vi "decimate cond.vi"(7 "Offset":i32, 8 "error in":errorcluster, 9 "B field array":dbl[](array[numeric]), 10 "Conductance":T1(graph), 11 "Decimation":i32) -> (0 "error out":errorcluster, 2 "decimated B field array":dbl[](array[numeric]), 3 "Decimated conductance":T1(graph))   [LabVIEW 2016, in "Tranconductance SM.lvclass"]
uses:
  Tranconductance SM.lvclass
  <userlib>/_MGI/1D Array/MGI Decimate Array with Offset/MGI Decimate Array with Offset (DBL[]).vi
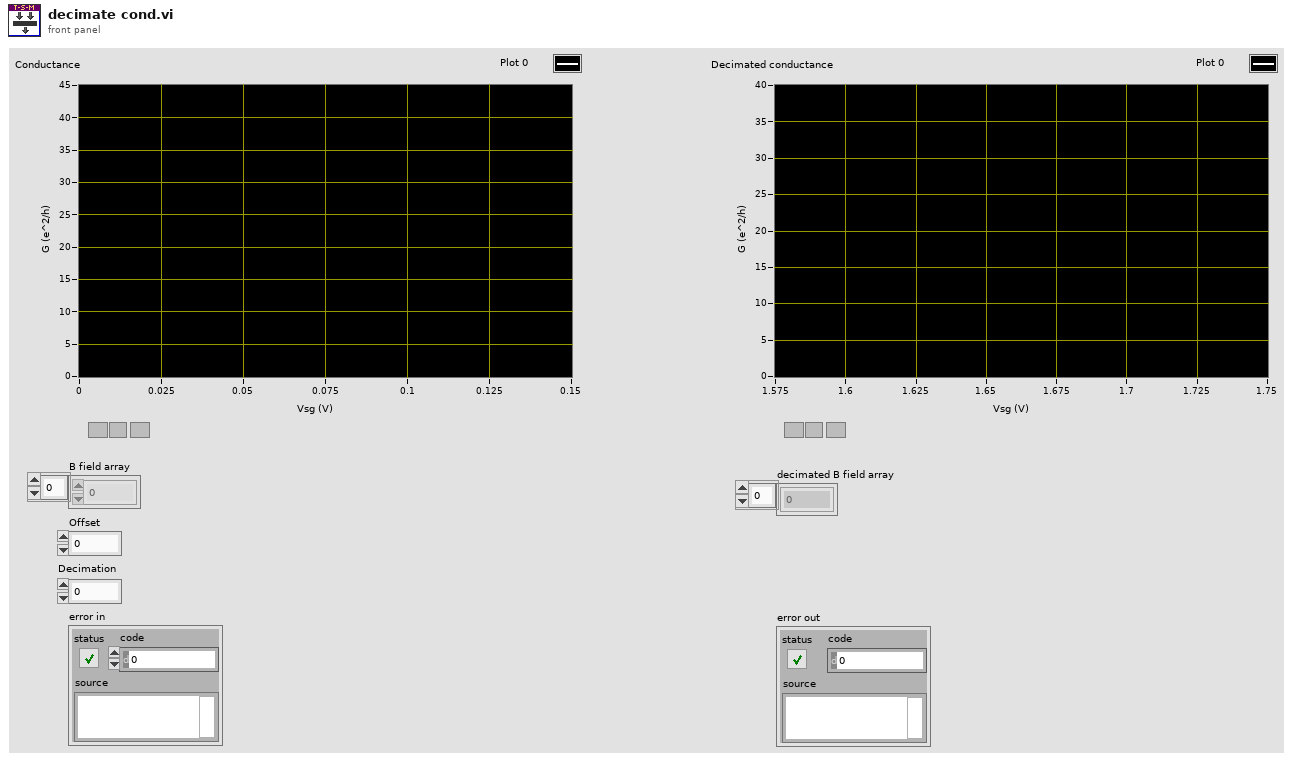
[diagram p1: front panel]
types:
  T1 = cluster{"Vfast":dbl[], "Decimated Array":dbl[]}[]
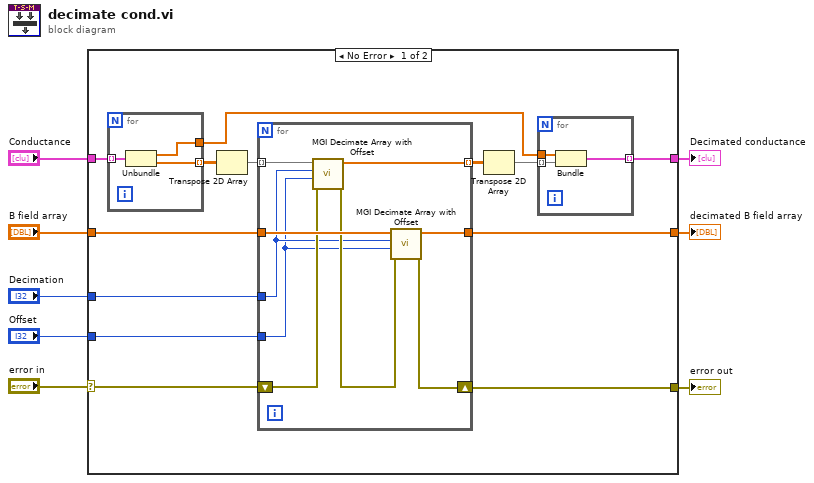
[diagram p0: block diagram]
diagram:
  n1 = case shown="No Error" "error in" {
    selector: "error in" -> [w11 w39]
    tunnel: "Conductance" -> [w21 w37]
    tunnel: [w16 w37] -> w7
    tunnel: "B field array" -> [w15 w38]
    tunnel: [w14 w38] -> w5
    tunnel: [w13 w39] -> w4
    tunnel: "Decimation" -> [w10 _]
    tunnel: "Offset" -> [w9 _]
    frame No Error {
      n2 = for {
        tunnel: w21 -> [w36] mode=indexing
        tunnel: [w35] -> w20 mode=indexing
        tunnel: [w34] -> w12
        n3 = Unbundle(w36) -> ("Vfast"=w34:dbl[], "Decimated Array"=w35:dbl[])
      }
      n4 = Transpose 2D Array(2D array=w20) -> (transposed array=w19:dbl[][])
      n5 = for {
        tunnel: w19 -> [w33] mode=indexing
        tunnel: [w32] -> w18 mode=indexing
        tunnel: w15 -> [w31]
        tunnel: [w30] -> w14
        shift-right: [w28] -> w13
        shift-left: w11 -> [w27]
        tunnel: w10 -> [w26]
        tunnel: w9 -> [w25]
        n6 = call-poly <userlib>:"MGI Decimate Array with Offset.vi"("error in (no error)"=w27, "Offset"=w25, "Decimation"=w26, "Double[] In"=w33) -> ("error out"=w29:errorcluster, "Double[] Out"=w32:dbl[])  [unwired: 6 in]
        n7 = call-poly <userlib>:"MGI Decimate Array with Offset.vi"("error in (no error)"=w29, "Offset"=w25, "Decimation"=w26, "Double[] In"=w31) -> ("error out"=w28:errorcluster, "Double[] Out"=w30:dbl[])  [unwired: 6 in]
      }
      n8 = Transpose 2D Array(2D array=w18) -> (transposed array=w17:dbl[][])
      n9 = for {
        tunnel: w17 -> [w24] mode=indexing
        tunnel: w12 -> [w23]
        tunnel: [w22] -> w16 mode=indexing
        n10 = Bundle("Vfast"=w23, w24) -> (w22:cluster{"Vfast":dbl[], dbl[]})  [unwired: 1 in]
      }
    }
    frame Error {
    }
  }
  "Decimated conductance" <- w7
  "decimated B field array" <- w5
  "error out" <- w4
